vi "logfile.vi"(8 "Error In":errorcluster, 9 "Locale":string="report.txt", 10 "Text In":string[](array[string]), 11 "Path In":path) -> (0 "Error Out":errorcluster, 3 "Path Out":path)   [LabVIEW 2014]
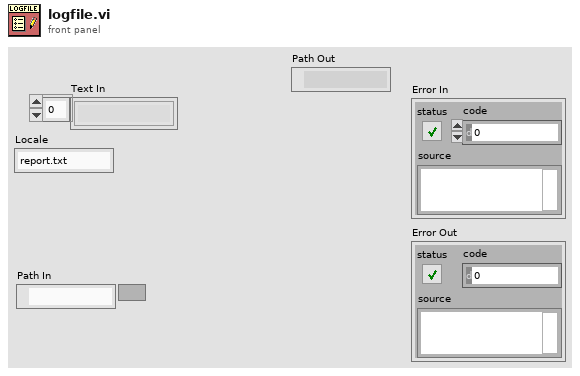
[diagram p1: front panel]
types:
  T1 = enum16{"open", "replace", "create", "open or create", "replace or create", "replace or create with confirmation"}
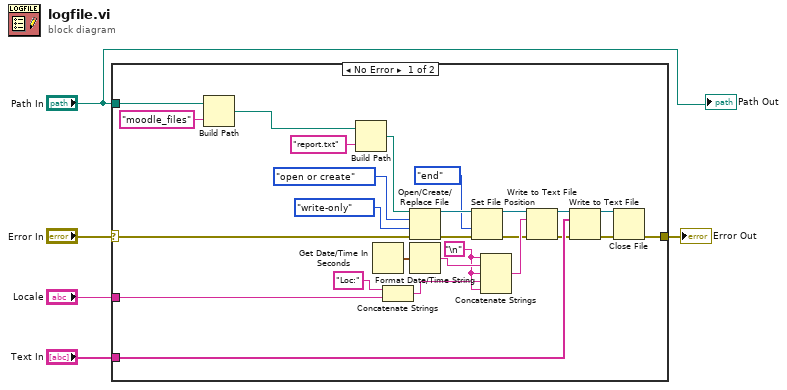
[diagram p0: block diagram]
diagram:
  n1 = case shown="No Error" "Error In" {
    selector: "Error In" -> [w26 w32]
    tunnel: "Text In" -> [w31 _]
    tunnel: "Path In" -> [w8 _]
    tunnel: [w20 w32] -> w3
    tunnel: "Locale" -> [w10 _]
    frame No Error {
      w12 = "\n"
      n2 = Build Path(base path=w8, name or relative path="moodle_files") -> (appended path=w6:path)
      n3 = Build Path(base path=w6, name or relative path="report.txt") -> (appended path=w29:path)
      n4 = Get Date/Time In Seconds() -> (seconds since 1Jan1904=w24:timestamp)
      n5 = Concatenate Strings("Loc:" ("string"), w10) -> (w11:string)
      n6 = Open/Create/Replace File(file path (use dialog)=w29, error in=w26, operation (0:open)=T1."open or create", access (0:read/write)=enum16{"read/write", "read-only", "write-only"}."write-only") -> (refnum out=w14:refnum<file>, error out=w17:errorcluster)  [unwired: 2 in, 1 out]
      n7 = Format Date/Time String(seconds (now)=w24) -> (date/time string=w23:string)  [unwired: 2 in]
      n8 = Set File Position(refnum=w14, from (0:start)=enum16{"start", "end", "current"}."end", error in=w17) -> (refnum out=w15:refnum<file>, error out=w16:errorcluster)  [unwired: 1 in]
      n9 = Concatenate Strings(w12, w23, w12, w11, w12) -> (w22:string)
      n10 = Write to Text File(file (use dialog)=w15, text=w22, error in=w16) -> (refnum out=w19:refnum<file>, error out=w25:errorcluster)  [unwired: 1 in, 1 out]
      n11 = Write to Text File(file (use dialog)=w19, text=w31, error in=w25) -> (refnum out=w18:refnum<file>, error out=w21:errorcluster)  [unwired: 1 in, 1 out]
      n12 = Close File(refnum=w18, error in=w21) -> (error out=w20:errorcluster)  [unwired: 1 out]
    }
    frame Error {
    }
  }
  "Error Out" <- w3
  "Path Out" <- "Path In"
